vi "Get_Do.vi"(0 "reference in":refnum<class "DO.lvclass">) -> (8 "DO":bool)   [LabVIEW 2019, in "DO.lvclass"]
uses:
  DO.lvclass
  DO.lvclass/DO.ctl
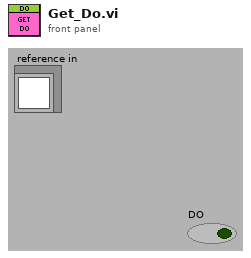
[diagram p1: front panel]
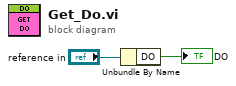
[diagram p0: block diagram]
diagram:
  n1 = Unbundle By Name("reference in") -> ("DO"=→"DO":bool)
